vi "Filename - Has Block Diagram.vi"(1 "Filename (including file extension)":string) -> (0 "Has Block Diagram?":bool)   [LabVIEW 2022 SP3]
doc: "Returns True if the input Filename is that of file that has a block diagram (i.e. a VI, not a CTL)"
panel:
  # "Development\ncontrols/indicators useful for development and testing, but which are not outputs of the VI"
  # "Input\nInputs to the VI"
  # "Output\nOutputs of the VI"
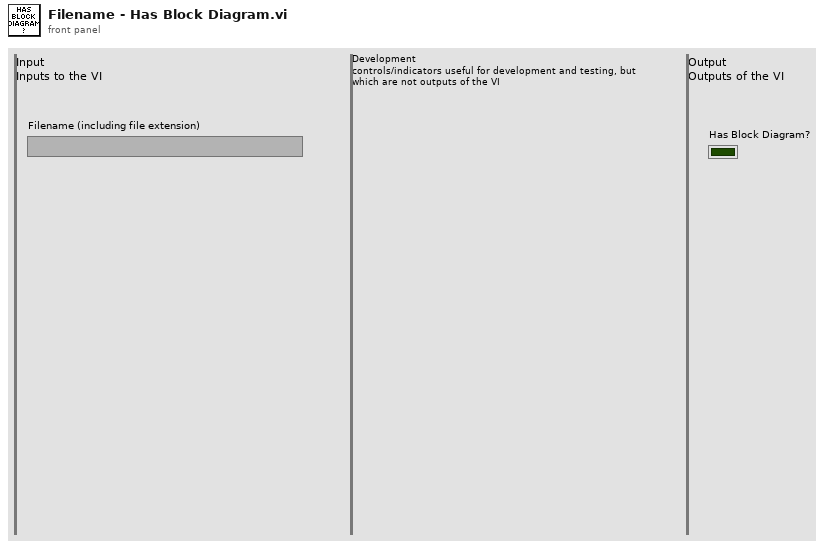
[diagram p1: front panel]
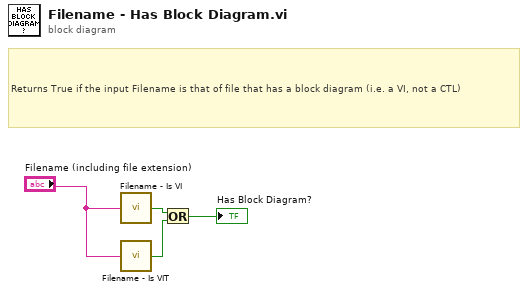
[diagram p0: block diagram]
diagram:
  # "Returns True if the input Filename is that of file that has a block diagram (i.e. a VI, not a CTL)"
  n1 = call "Filename - Is VI.vi"("Filename (including file extension)"="Filename (including file extension)") -> ("Is VI?"=w3:bool)
  n2 = call "Filename - Is VIT.vi"("Filename (including file extension)"="Filename (including file extension)") -> ("Is VIT?"=w4:bool)
  n3 = Or(x=w3, y=w4) -> (x .or. y?=→"Has Block Diagram?":bool)
